vi "ValidIPAddr.vi"(11 "IP Address String":string="192.168.0.1") -> (0 "error out":errorcluster, 2 "return type":i32, 3 "IP Address String out":string="192.168.0.1")   [LabVIEW 2017, in "Shared Variables CD 2.0 Configuration.lvlib"]
doc: "0 invalid IP address\n1 valid IP address"
uses:
  Shared Variables CD 2.0 Configuration.lvlib
  ws2_32.dll
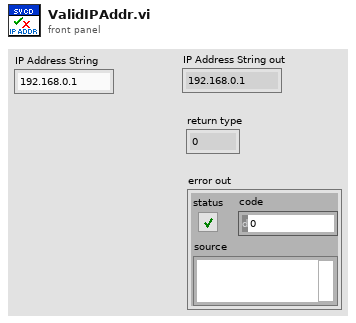
[diagram p1: front panel]
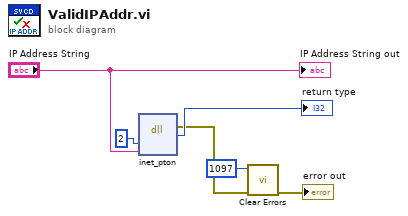
[diagram p0: block diagram]
diagram:
  n1 = dll-call lib="ws2_32.dll" fn="inet_pton"("Family"=2, "pszAddrString"="IP Address String") -> (error out=w2:errorcluster, "return type"=→"return type":i32)  [unwired: 5 in, 1 out]
  n2 = call <vilib>:"Clear Errors.vi"("error in (no error)"=w2, "specific error code to clear (0: all)"=1097) -> ("error out"=→"error out":errorcluster)  [unwired: 4 in, 1 out]
  "IP Address String out" <- "IP Address String"
